vi "nipkg-createPackageControlFile.vi"(8 "error in (no error)":errorcluster, 11 "Package directory":path) -> (0 "error out":errorcluster, 3 "Package directory out":path)   [LabVIEW 2014, in "nipkg-build-system.lvlib"]
uses:
  nipkg-build-system.lvlib
  types/Package Metadata string constants.ctl
  <vilib>/Utility/file.llb/Write To Spreadsheet File (string).vi
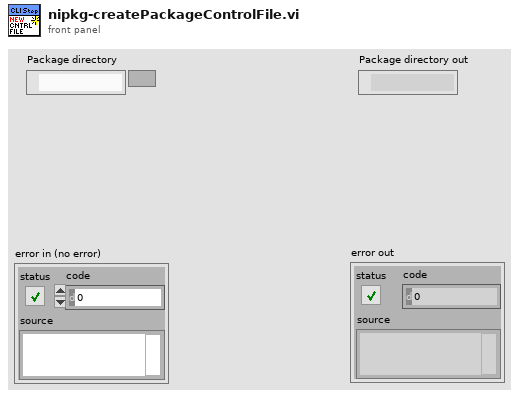
[diagram p1: front panel]
types:
  T1 = typedef "nipkg-build-system.lvlib/Package Metadata string constants.ctl" = string[]
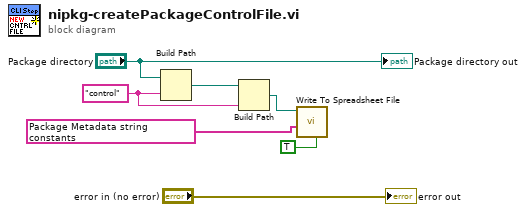
[diagram p0: block diagram]
diagram:
  w3 = "control" ("name or relative path")
  n1 = Build Path(base path="Package directory", name or relative path=w3) -> (appended path=w4:path)
  n2 = Build Path(base path=w4, name or relative path=w3) -> (appended path=w2:path)
  n3 = call-poly <vilib>:"Write To Spreadsheet File.vi"("transpose? (no:F)"=TRUE, "1D data"=T1 ["Package: waveform-processing-custom-device-2017", "Version: 1.0.0.0", "Architecture: windows_x64", "Maintainer: Absolutely no one.", "XB-Plugin: file", "Description: Pretty cool package.", "XB-Eula:  ", "Priority: standard", "Homepage: http://www.ni.com", "XB-LanguageSupport: en", "Section: Infrastructure", "XB-DisplayVersion: 1.0.0", "XB-DisplayName: Waveform Processing Custom Device 2017", "Depends: "] ("NIPM Package Metadata Fields Constant"), "file path (dialog if empty)"=w2) -> ()  [unwired: 5 in, 1 out]
  "error out" <- "error in (no error)"
  "Package directory out" <- "Package directory"
